vi "Base Init.vi"(6 "Creator":refnum<user-event>, 8 "Creator Alias":string, 9 "Self":refnum<user-event>, 10 "Self Alias":string) -> (2 "Addresses Strategy out":refnum<class "Addresses Strategy.lvclass">)   [LabVIEW 2021, in "jettl.lvlib" / "Addresses Strategy.lvlib"]
uses:
  Addresses Strategy.lvlib
  Addresses Strategy/Addresses Strategy.lvclass
  Msg/Msg.lvclass
  Base Addresses Strategy/Base Addresses Strategy.lvclass
  C:/git/jettl/jettl/jettl/Addresses Strategy/Addresses Strategy/Addresses Strategy.lvclass
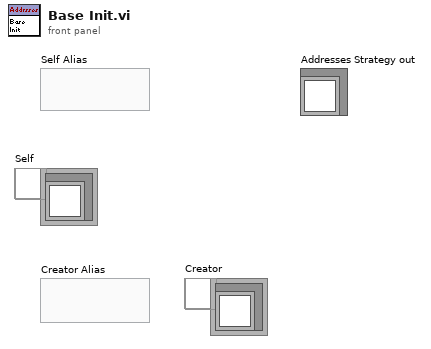
[diagram p1: front panel]
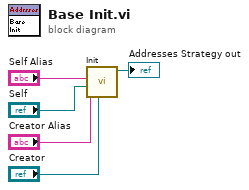
[diagram p0: block diagram]
diagram:
  n1 = call "Init.vi"("Creator"="Creator", "Creator Alias"="Creator Alias", "Self"="Self", "Self Alias"="Self Alias") -> ("Base Addresses Strategy out"=→"Addresses Strategy out":refnum<class "Base Addresses Strategy.lvclass">)  [unwired: 7 in]
